vi "ex5-7.vi"   [LabVIEW 2014]
uses:
  <vilib>/NXT/Subs/MotorOutput.ctl
  <vilib>/NXT/Block Support/NXT_ButtonSelector.ctl
  <vilib>/NXT/Dual Mode Library/Motors/MotorOn.vi
  <vilib>/NXT/Dual Mode Library/Waits/Wait_Num.vi
  <vilib>/NXT/Dual Mode Library/Sensors/readNXTButton.vi
  <vilib>/NXT/Dual Mode Library/Motors/MotorBrake.vi
types:
  T1 = typedef "MotorOutput.ctl" = u8
  T2 = typedef "LVHSConnector.ctl" = refnum<class "BrickReference.lvclass">
  T3 = typedef "NXT_ButtonSelector.ctl" = u16
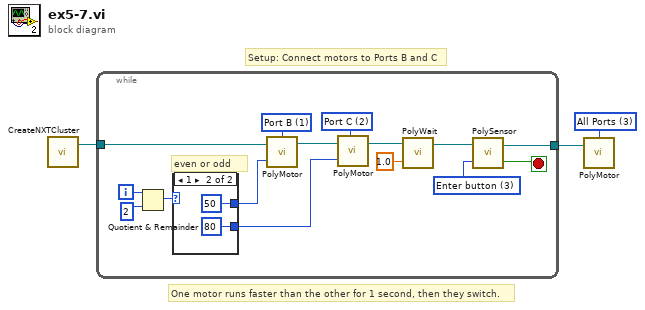
[diagram p0: block diagram]
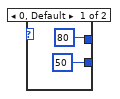
[diagram p2: hidden frame]
diagram:
  w2 = T1 3 items=["Port A", "Port B", "Port C", "All Ports"] ("Output Port")
  # "Setup: Connect motors to Ports B and C"
  # "One motor runs faster than the other for 1 second, then they switch."
  n1 = call <vilib>:"CreateNXTCluster.vi"() -> ("NXT/EV3"=w3:T2)  [unwired: 4 in]
  n2 = while {
    tunnel: w3 -> [w14]
    tunnel: [w7] -> w1
    i -> [w10]
    stop <- w6 stop-if-true
    w5 = T3 3 items=["Enter button"=3, "Left button"=2, "Right button"=1] ("Button (Enter button)")
    w15 = T1 2 items=["Port A", "Port B", "Port C", "All Ports"] ("Output Port")
    w16 = T1 1 items=["Port A", "Port B", "Port C", "All Ports"] ("Output Port")
    # "even or odd"
    n3 = Quotient & Remainder(x=w10, y=2) -> (x-y*floor(x/y)=w9:i32)  [unwired: 1 out]
    n4 = case shown="1" w9 {
      tunnel: [80 50] -> w8
      tunnel: [50 80] -> w4
      frame 0, Default {
      }
      frame 1 {
      }
    }
    n5 = call-poly <vilib>:"PolyMotor.vi"("Power (75)"=w8, "NXT/EV3"=w14, "Output Port (All Ports)"=w16) -> ("NXT/EV3"=w17:T2)  [unwired: 1 out]
    n6 = call-poly <vilib>:"PolyMotor.vi"("Power (75)"=w4, "NXT/EV3"=w17, "Output Port (All Ports)"=w15) -> ("NXT/EV3"=w12:T2)  [unwired: 1 out]
    n7 = call-poly <vilib>:"PolyWait.vi"("Time (1 sec)"=sgl 1.0 ("Time (sec)"), "NXT/EV3"=w12) -> ("NXT/EV3"=w11:T2)  [unwired: 2 out]
    n8 = call-poly <vilib>:"PolySensor.vi"("Button (Enter button)"=w5, "NXT/EV3"=w11) -> ("Yes/No"=w6:bool, "NXT/EV3"=w7:T2)  [unwired: 1 out]
  }
  n9 = call-poly <vilib>:"PolyMotor.vi"("NXT/EV3"=w1, "Port (All Ports)"=w2) -> ()  [unwired: 3 out]
